vi "Add Result.vi"(8 "error in (no error)":errorcluster, 9 "Add in front":bool, 10 "Results to add":refnum<class "Acquired Result.lvclass">[](array[class]), 11 "Combined Result in":refnum<class "Combined Result.lvclass">) -> (0 "error out":errorcluster, 3 "Combined Result out":refnum<class "Combined Result.lvclass">)   [LabVIEW 2021, in "Combined Result.lvclass"]
uses:
  Combined Result.lvclass
  Acquired Result/Acquired Result.lvclass
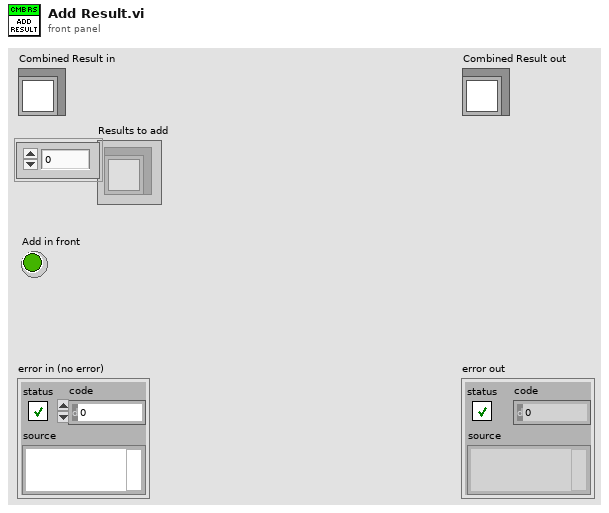
[diagram p1: front panel]
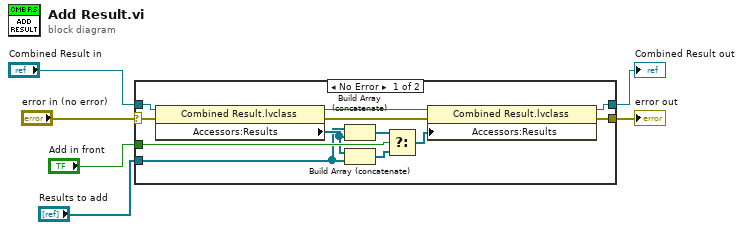
[diagram p0: block diagram]
diagram:
  n1 = case shown="No Error" "error in (no error)" {
    selector: "error in (no error)" -> [w18 w20]
    tunnel: [w15 w20] -> w5
    tunnel: [w13 w19] -> w3
    tunnel: "Combined Result in" -> [w16 w19]
    tunnel: "Add in front" -> [w11 _]
    tunnel: "Results to add" -> [w8 _]
    frame No Error {
      n2 = property class="Combined Result.lvclass"(reference=w16, error in=w18) -> (reference out=w14:refnum<class "Combined Result.lvclass">, error out=w17:errorcluster, "Accessors:Results"=w9:refnum<class "Acquired Result.lvclass">[])
      n3 = Build Array (concatenate)(w8, w9) -> (w10:refnum<class "Acquired Result.lvclass">[])
      n4 = Build Array (concatenate)(w9, w8) -> (w7:refnum<class "Acquired Result.lvclass">[])
      n5 = Select(t=w10, s=w11, f=w7) -> (s? t:f=w12:refnum<class "Acquired Result.lvclass">[])
      n6 = property class="Combined Result.lvclass"(reference=w14, error in=w17, "Accessors:Results"=w12) -> (reference out=w13:refnum<class "Combined Result.lvclass">, error out=w15:errorcluster)
    }
    frame Error {
    }
  }
  "error out" <- w5
  "Combined Result out" <- w3
